vi "user initialization.vi"(8 "error in":errorcluster, 10 "configuration in":refnum<class "control module configuration.lvclass">, 11 "System Diagnostics runtime in":refnum<class "System Diagnostics runtime.lvclass">) -> (0 "error out":errorcluster, 3 "System Diagnostics runtime out":refnum<class "System Diagnostics runtime.lvclass">)   [LabVIEW 2013, in "System Diagnostics runtime.lvclass"]
uses:
  System Diagnostics runtime.lvclass
  <vilib>/NI/DCAF/Tag Editor Core/control module/configuration/control module configuration.lvclass
  configuration/System Diagnostics configuration.lvclass
  <vilib>/NI/DCAF/Tag Editor Core/control module/runtime/control module runtime.lvclass
  System Diagnostics runtime.lvclass/System Diagnostics runtime.ctl
  <vilib>/nisyscfg/nisyscfg.lvlib
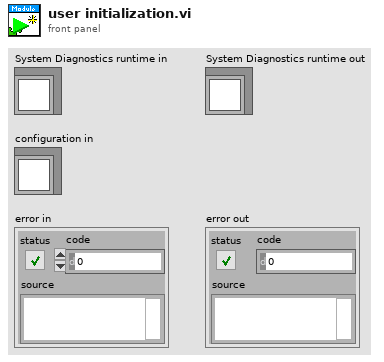
[diagram p1: front panel]
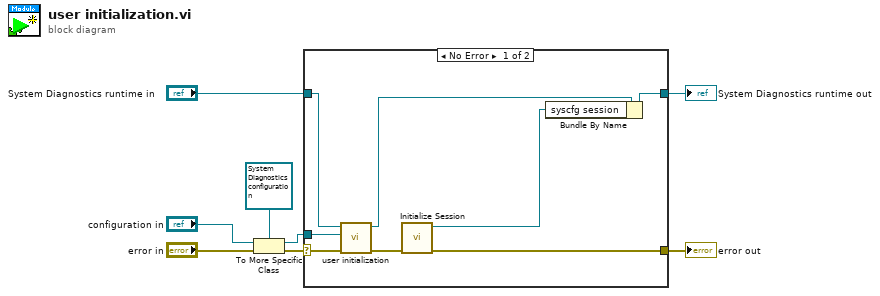
[diagram p0: block diagram]
diagram:
  n1 = To More Specific Class(target class=refnum<class "System Diagnostics configuration.lvclass"> refnum ("user module configuration"), reference="configuration in", error in="error in") -> (specific class reference=w1:refnum<class "System Diagnostics configuration.lvclass">, error out=w5:errorcluster)
  n2 = case shown="No Error" w5 {
    selector: w5 -> [w15 w17]
    tunnel: [w16 w18] -> w4
    tunnel: "System Diagnostics runtime in" -> [w11 w18]
    tunnel: [w14 w17] -> w3
    tunnel: w1 -> [w9 _]
    frame No Error {
      n3 = call-parent "user initialization.vi"("error in"=w15, "configuration in"=w9, "fixed channel runtime in"=w11) -> ("error out"=w12:errorcluster, "fixed channel runtime out"=w10:refnum<class "System Diagnostics runtime.lvclass">)  [unwired: 7 in]
      n4 = call <vilib>:"Initialize Session.vi"("error in (no error)"=w12) -> ("error out"=w14:errorcluster, "Session out"=w13:refnum<k21>)  [unwired: 9 in]
      n5 = Bundle By Name(cluster=w10, "syscfg session"=w13) -> (w16:refnum<class "System Diagnostics runtime.lvclass">)
    }
    frame Error {
    }
  }
  "error out" <- w3
  "System Diagnostics runtime out" <- w4
